vi "SubVI.vi"(1 "Delay Time (s)":dbl=1.0, 2 "Nivel de entrada":dbl) -> (0 "Waveform Chart":dbl(graph))   [LabVIEW 2015]
panel:
  # "Generador de señales"
  # "Serrano Bermúdez Luis Esteban\nFecha de Entrega 17/02/2019"
  # "Descripción: Esta aplicacion crea un generador de señales aleatorias cada segundo.\nEsta aplicacion es diseñada para poder funcionar dentro de otra aplicacion de LabVIEW\ncomo un subVI"
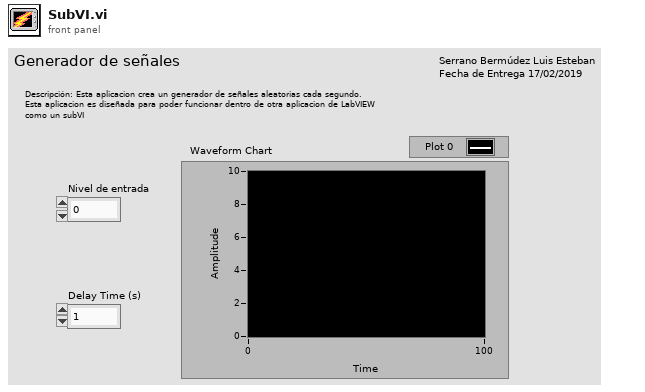
[diagram p1: front panel]
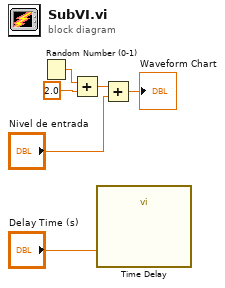
[diagram p0: block diagram]
diagram:
  n1 = Random Number (0-1)() -> (number: 0 to 1=w5:dbl)
  n2 = Add(x=w5, y=2.0) -> (x+y=w4:dbl)
  n3 = call "Time Delay"("Delay Time (s)"="Delay Time (s)") -> ()  [unwired: 10 in, 1 out]
  n4 = Add(x=w4, y="Nivel de entrada") -> (x+y=→"Waveform Chart":dbl)
